vi "POST File.vi"(6 "timeout (10000)":i32=10000, 7 "output file":path=path "", 8 "error in (no error)":errorcluster, 9 "file":path, 10 "url":string, 11 "HTTP Client Abstract in":refnum<class "HTTP Client reqwest.lvclass">) -> (0 "error out":errorcluster, 1 "body":string, 2 "headers":string, 3 "HTTP Client Abstract out":refnum<class "HTTP Client reqwest.lvclass">, 4 "status code":u32)   [LabVIEW 2020, in "HTTP Client reqwest.lvclass"]
uses:
  HTTP Client reqwest.lvclass
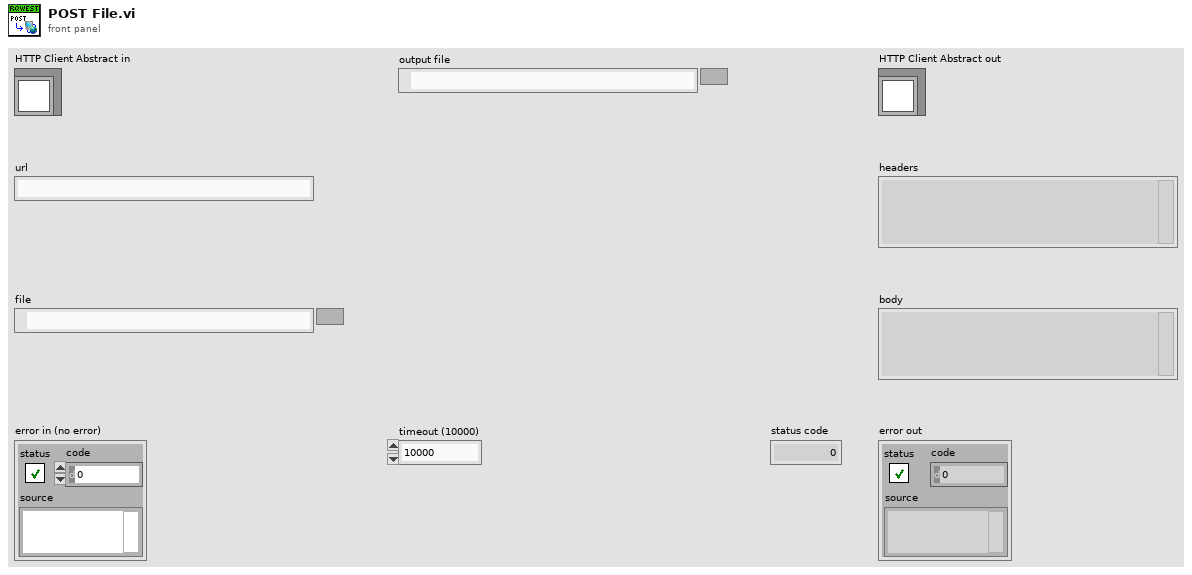
[diagram p1: front panel]
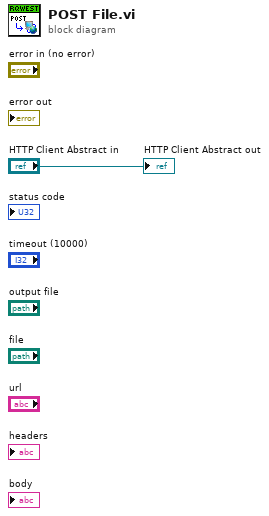
[diagram p0: block diagram]
diagram:
  "HTTP Client Abstract out" <- "HTTP Client Abstract in"
